vi "Debugging globals.vi"() -> ()   [LabVIEW 2019]
doc: "Used to enable and disable tracing. You may want to place other debugging control elements here."
panel:
  in  "Tracing":bool
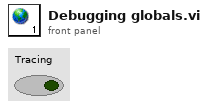
[diagram p1: front panel]
diagram:
